vi "Extract Line.vi"(0 "image in":refnum<class "MSC Image.lvclass">, 1 "Line Points":T1, 2 "Connectivity":T2=4 items=["4-connected"=4, "8-connected"=8], 5 "error in (no error)":errorcluster) -> (14 "image out":refnum<class "MSC Image.lvclass">, 15 "Extracted Line Profile":dbl[](array[numeric]), 16 "Line Length":u32, 19 "error out":errorcluster)   [LabVIEW 2016, in "MSC Image.lvclass"]
doc: "Extracts a line profile from an image."
uses:
  MSC Image.lvclass
  Dependencies/x86/MSC I Process32.dll
  controls/Line Connectivity.ctl
  controls/Contour.ctl
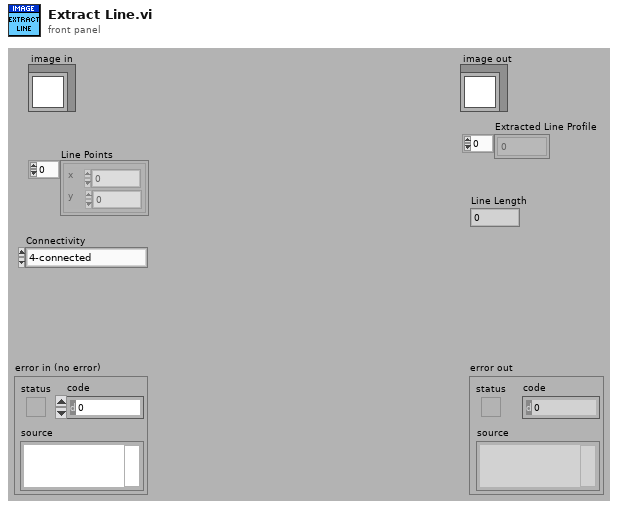
[diagram p1: front panel]
types:
  T1 = typedef "MSC Image.lvclass/Contour.ctl" = cluster{"x":i16, "y":i16}[]
  T2 = typedef "MSC Image.lvclass/Line Connectivity.ctl" = u16
  T3 = typedef "Image.ctl" = cluster{"Pointer":u64, "Size":T4, "Image Type":T5, "Time Stamp":timestamp, "Variant":variant}
  T4 = typedef "Size.ctl" = cluster{"Cols":i32, "Rows":i32}
  T5 = typedef "Image Type.ctl" = i32
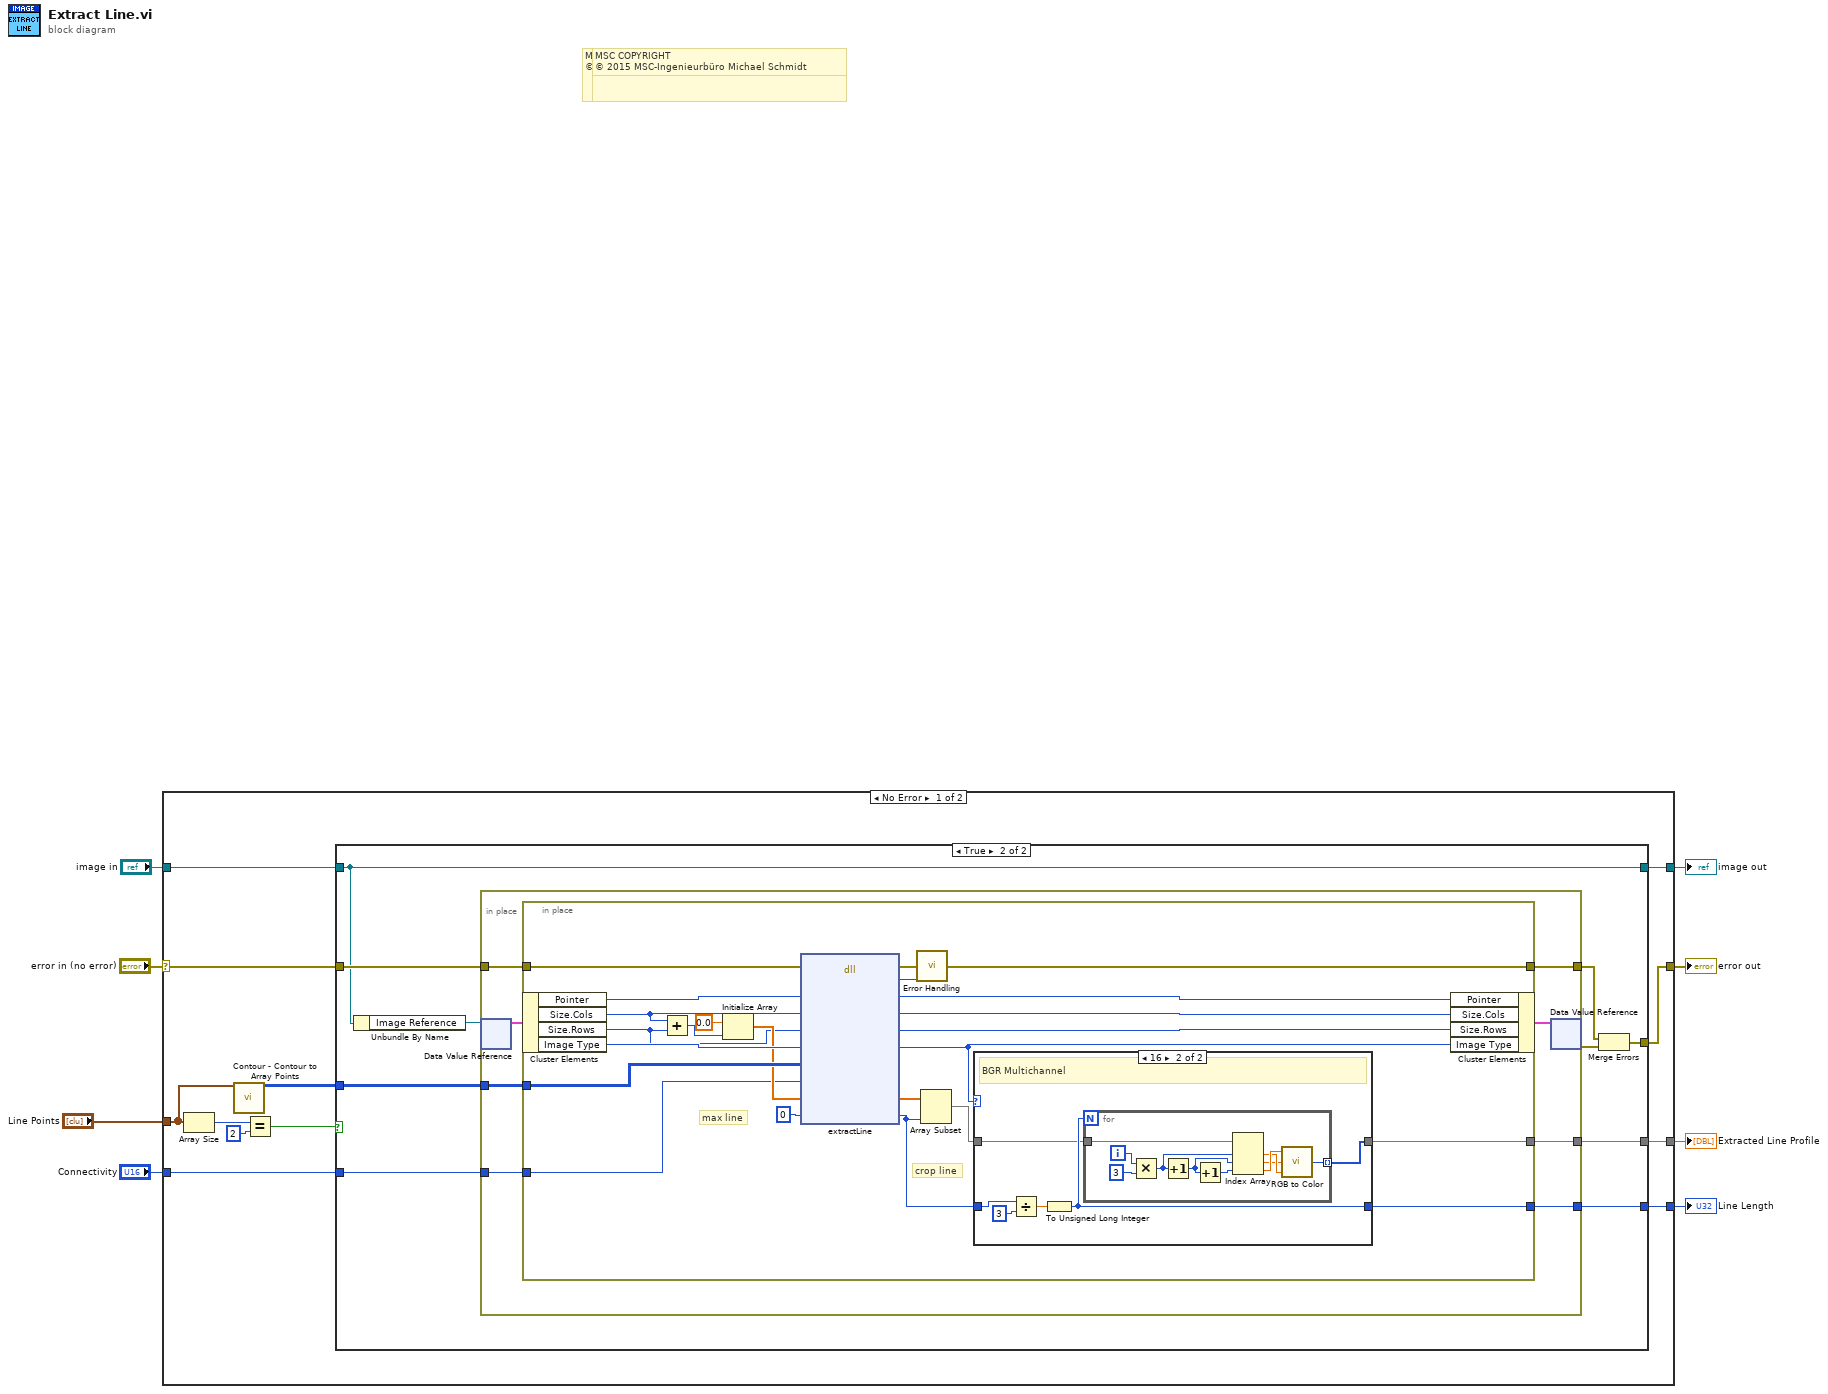
[diagram p0: block diagram]
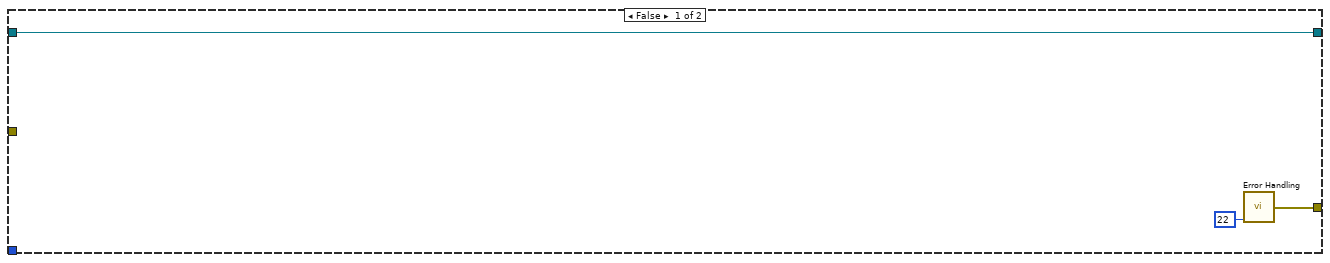
[diagram p2: hidden frame]
diagram:
  # "MSC COPYRIGHT\n© 2016 MSC-Ingenieurbüro Michael Schmidt"
  # "MSC COPYRIGHT\n© 2016 MSC-Ingenieurbüro Michael Schmidt"
  # "MSC COPYRIGHT\n© 2015 MSC-Ingenieurbüro Michael Schmidt"
  # "MSC COPYRIGHT\n© 2015 MSC-Ingenieurbüro Michael Schmidt"
  n1 = case shown="No Error" "error in (no error)" {
    selector: "error in (no error)" -> [w10 w83]
    tunnel: [w20 w83] -> w6
    tunnel: [w17 _] -> w2
    tunnel: "Connectivity" -> [w16 _]
    tunnel: "Line Points" -> [w14 _]
    tunnel: "image in" -> [w12 w84]
    tunnel: [w11 w84] -> w3
    tunnel: [w9 _] -> w1
    frame No Error {
      n2 = Array Size(array=w14) -> (size(s)=w15:i32)
      n3 = call "Contour - Contour to Array Points.vi"("Contour"=w14) -> ("Array Points"=w13:i16[][])  [unwired: 14 in]
      n4 = Equal?(x=w15, y=2) -> (x = y?=w18:bool)
      n5 = case shown="True" w18 {
        tunnel: w10 -> [_ w31]
        tunnel: [w21 w30] -> w20
        tunnel: w13 -> [_ w29]
        tunnel: [_ w28] -> w9
        tunnel: [_ w27] -> w17
        tunnel: w16 -> [_ w26]
        tunnel: w12 -> [w23 w24]
        tunnel: [w23 w24] -> w11
        frame False {
          n6 = call "Error Handling.vi"("return type"=22) -> ("error out"=w21:errorcluster)  [unwired: 13 in, 1 out]
        }
        frame True {
          n7 = Unbundle By Name(w24) -> ("Image Reference"=w25:refnum<data-value>)
          n8 = in-place {
            in-place-border: w31 -> [w39]
            in-place-border: [w38] -> w32
            in-place-border: w29 -> [w37]
            in-place-border: [w36] -> w28
            in-place-border: [w35] -> w27
            in-place-border: w26 -> [w34]
            n9 = in-place-dvr #1(w25) -> (w40:T3)  [unwired: 1 out]
            n10 = in-place {
              in-place-border: w39 -> [w59]
              in-place-border: [w64] -> w38
              in-place-border: w37 -> [w55]
              in-place-border: [w49] -> w36
              in-place-border: [w47] -> w35
              in-place-border: w34 -> [w45]
              # "crop line"
              # "max line"
              n11 = in-place-cluster #2(w40) -> ("Pointer"=w63:u64, "Size.Cols"=w44:i32, "Size.Rows"=w43:i32, "Image Type"=w56:T5)
              n12 = Add(x=w44, y=w43) -> (x+y=w42:i32)
              n13 = Initialize Array(0.0, w42) -> (w53:dbl[])
              n14 = dll-call lib="C:/Users/MSC/LabVIEW Projekte/LV 2014/MSC I-Process/user.lib/MSC-I Process/Dependencies/x86/MSC I Process*.dll" fn="extractLine"(error in=w59, "pointer"=w63, "cols"=w44, "rows"=w43, "type"=w56, "points"=w55, "connectivity"=w45, "line"=w53, "lineLength"=0) -> (error out=w58:errorcluster, "error"=w57:i32, "pointer"=w62:u64, "cols"=w61:i32, "rows"=w60:i32, "type"=w50:i32, "line"=w51:dbl[], "lineLength"=w46:i32)  [unwired: 4 in, 1 out]
              n15 = call "Error Handling.vi"("error in (no error)"=w58, "return type"=w57) -> ("error out"=w64:errorcluster)  [unwired: 12 in, 1 out]
              n16 = Array Subset(array=w51, length=w46) -> (w48:dbl[])  [unwired: 1 in]
              n17 = case shown="16" w50 {
                tunnel: [w65 w67] -> w49
                tunnel: w48 -> [w65 w68]
                tunnel: [w66 w69] -> w47
                tunnel: w46 -> [w66 w72]
                frame Default {
                }
                frame 16 {
                  # "BGR Multichannel"
                  n18 = Divide(x=w72, y=3) -> (x/y=w70:dbl)
                  n19 = To Unsigned Long Integer(number=w70) -> (unsigned 32bit integer=w69:u32)
                  n20 = for {
                    N: w69 -> [_]
                    tunnel: w68 -> [w81]
                    tunnel: [w77] -> w67 mode=indexing
                    i -> [w76]
                    n21 = Multiply(x=w76, y=3) -> (x*y=w80:i32)
                    n22 = Increment(x=w80) -> (x+1=w79:i32)
                    n23 = Increment(x=w79) -> (x+1=w78:i32)
                    n24 = Index Array(array=w81, index #1=w80, index #2=w79, index #3=w78) -> (element #1=w74:dbl, element #2=w73:dbl, element #3=w75:dbl)
                    n25 = call <vilib>:"RGB to Color.vi"("B"=w74, "G"=w73, "R"=w75) -> ("Color"=w77:u32)
                  }
                }
              }
              n26 = in-place-cluster #2("Pointer"=w62, "Size.Cols"=w61, "Size.Rows"=w60, "Image Type"=w50) -> (w41:T3)
            }
            n27 = in-place-dvr #1(w41) -> (w33:errorcluster)  [unwired: 1 out]
          }
          n28 = Merge Errors(w32, w33) -> (w30:errorcluster)
        }
      }
    }
    frame Error {
    }
  }
  "error out" <- w6
  "image out" <- w3
  "Line Length" <- w2
  "Extracted Line Profile" <- w1
